vi "E-Cal and Port Extend.vi"(0 "ENA Visa Name":refnum<visa-resource-name>="E5080A", 11 "error in (no error)":errorcluster) -> (15 "error out":errorcluster)   [LabVIEW 2013]
panel:
  # "Press the Run button to start Calibration"
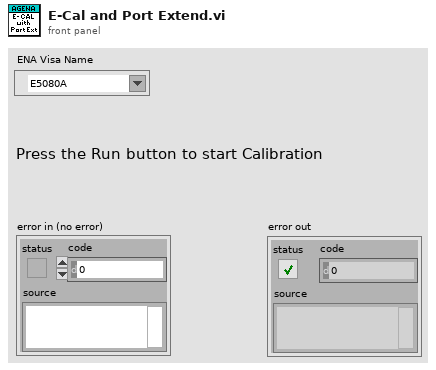
[diagram p1: front panel]
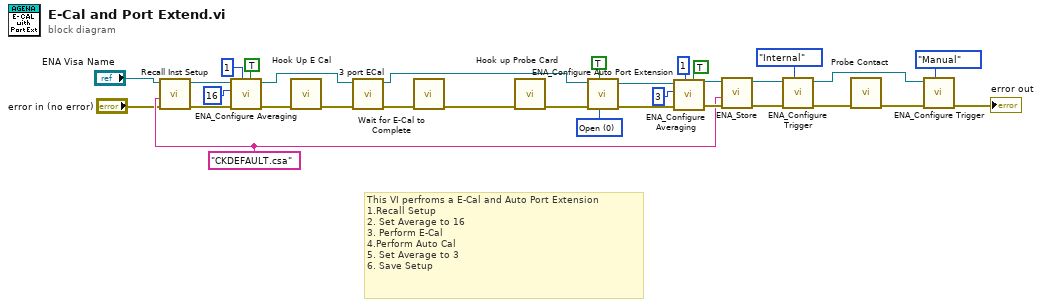
[diagram p0: block diagram]
diagram:
  w25 = 0 items=["Open", "Short"] ("Standard (1: Short)")
  w16 = "CKDEFAULT.csa" ("File Name ()")
  # "This VI perfroms a E-Cal and Auto Port Extension \n1.Recall Setup\n2. Set Average to 16\n3. Perform E-Cal\n4.Perform Auto Cal\n5. Set Average to 3\n6. Save Setup"
  n1 = call "Recall Inst Setup.vi"("error in (no error)"="error in (no error)", "File Name ()"=w16, "VISA resource name"="ENA Visa Name") -> ("error out"=w32:errorcluster, "VISA resource name out"=w31:refnum<visa-resource-name>)  [unwired: 7 in]
  n2 = call "ENA_Configure Averaging.vi"("Averaging State (F: Off)"=TRUE, "Channel (1)"=1, "error in (no error)"=w32, "Factor (16)"=16, "VISA resource name"=w31) -> ("error out"=w27:errorcluster, "VISA resource name out"=w12:refnum<visa-resource-name>)  [unwired: 5 in]
  n3 = call "Hook Up E Cal"("error in (no error)"=w27) -> ("error out"=w13:errorcluster)  [unwired: 9 in, 1 out]
  n4 = call "3 port ECal.vi"("error in (no error)"=w13, "VISA resource name"=w12) -> ("error out"=w10:errorcluster, "VISA resource name out"=w11:refnum<visa-resource-name>)  [unwired: 8 in]
  n5 = call "Wait for E-Cal to Complete"("error in (no error)"=w10) -> ("error out"=w9:errorcluster)  [unwired: 9 in, 1 out]
  n6 = call "Hook up Probe Card"("error in (no error)"=w9) -> ("error out"=w24:errorcluster)  [unwired: 9 in, 1 out]
  n7 = call "ENA_Configure Auto Port Extension.vi"("Standard (1: Short)"=w25, "Enable Auto Port Extension (T: Enable)"=TRUE, "error in (no error)"=w24, "VISA resource name"=w11) -> ("error out"=w20:errorcluster, "VISA resource name out"=w21:refnum<visa-resource-name>)  [unwired: 6 in]
  n8 = call "ENA_Configure Averaging.vi"("Averaging State (F: Off)"=TRUE, "Channel (1)"=1, "error in (no error)"=w20, "Factor (16)"=3, "VISA resource name"=w21) -> ("error out"=w18:errorcluster, "VISA resource name out"=w17:refnum<visa-resource-name>)  [unwired: 5 in]
  n9 = call "ENA_Store.vi"("error in (no error)"=w18, "File Name ()"=w16, "VISA resource name"=w17) -> ("error out"=w8:errorcluster, "VISA resource name out"=w6:refnum<visa-resource-name>)  [unwired: 7 in]
  n10 = call "ENA_Configure Trigger.vi"("Trigger Type"=enum16{"Internal", "Manual", "External"}."Internal", "error in (no error)"=w8, "VISA resource name"=w6) -> ("error out"=w7:errorcluster, "VISA resource name out"=w3:refnum<visa-resource-name>)  [unwired: 7 in]
  n11 = call "Probe Contact"("error in (no error)"=w7) -> ("error out"=w4:errorcluster)  [unwired: 9 in, 1 out]
  n12 = call "ENA_Configure Trigger.vi"("Trigger Type"=enum16{"Internal", "Manual", "External"}."Manual", "error in (no error)"=w4, "VISA resource name"=w3) -> ("error out"=→"error out":errorcluster)  [unwired: 7 in, 1 out]
